vi "ExcelLoop.vi"() -> ()   [LabVIEW 2017]
uses:
  <vilib>/Utility/file.llb/Read Delimited Spreadsheet (DBL).vi
panel:
  in  "disabled index (row) 3":i32
  in  "disabled index (row) 2":i32
  in  "disabled index (row)":i32
  out "Time":i32
  out "Numeric 6":i32
  out "Numeric 5":i32
  out "Numeric 4":i32
  out "Z Position":i32
  out "X Position":i32
  out "Y Position":i32
  out "Speed Z":i32
  out "Speed X":i32
  out "Speed Y":i32
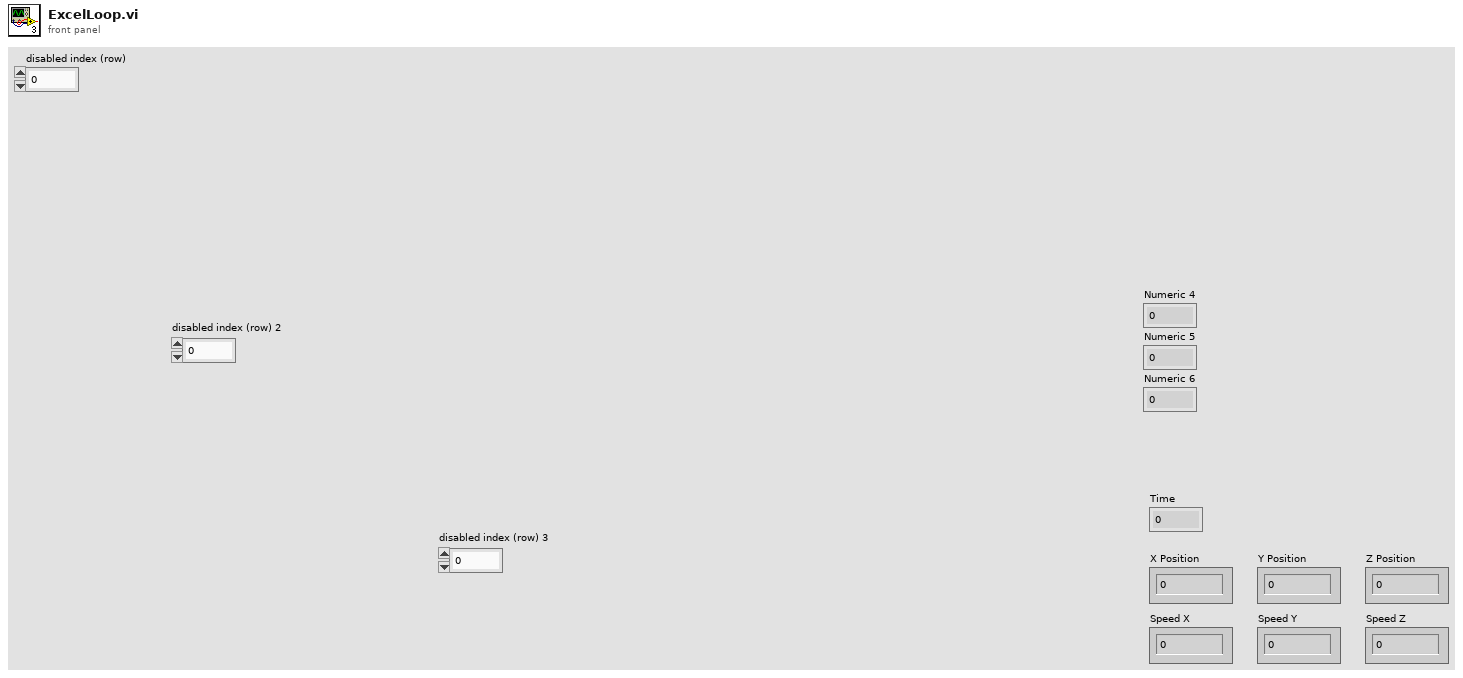
[diagram p1: front panel]
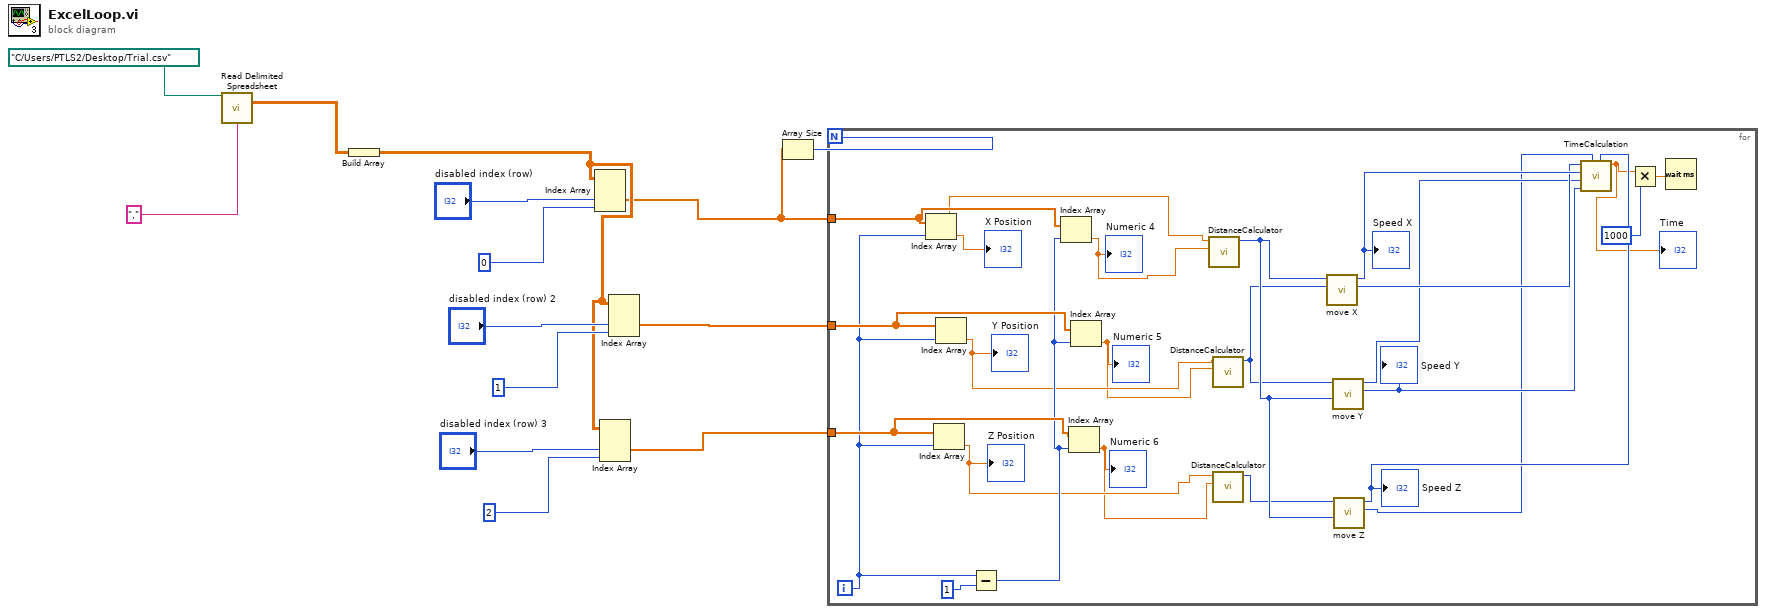
[diagram p0: block diagram]
diagram:
  n1 = call-poly <vilib>:"Read Delimited Spreadsheet.vi"("file path (dialog if empty)"=path "C:/Users/PTLS2/Desktop/Trial.csv", "delimiter (\\t)"="," ("delimiter (\\t)")) -> ("all rows"=w11:dbl[][])  [unwired: 8 in, 5 out]
  n2 = Build Array(w11) -> (w4:dbl[][][])
  n3 = Index Array(array=w4, index (dim 1)="disabled index (row)", index (dim 2)=0 ("disabled index (col)")) -> (element=w3:dbl[])  [unwired: 1 in]
  n4 = Index Array(array=w4, index (dim 1)="disabled index (row) 3", index (dim 2)=2 ("disabled index (col)")) -> (element=w1:dbl[])  [unwired: 1 in]
  n5 = Index Array(array=w4, index (dim 1)="disabled index (row) 2", index (dim 2)=1 ("disabled index (col)")) -> (element=w2:dbl[])  [unwired: 1 in]
  n6 = Array Size(array=w3) -> (size(s)=w14:i32)
  n7 = for {
    N: w14 -> [_]
    tunnel: w3 -> [w30]
    tunnel: w2 -> [w31]
    tunnel: w1 -> [w32]
    i -> [w24]
    n8 = Index Array(array=w30, index=w24) -> (element=w23:dbl)
    "X Position" <- w23
    n9 = Index Array(array=w32, index=w24) -> (element=w18:dbl)
    "Z Position" <- w18
    n10 = Index Array(array=w31, index=w24) -> (element=w20:dbl)
    "Y Position" <- w20
    n11 = Subtract(x=w24, y=1) -> (x-y=w25:i32)
    n12 = Index Array(array=w30, index=w25) -> (element=w22:dbl)
    "Numeric 4" <- w22
    n13 = Index Array(array=w32, index=w25) -> (element=w17:dbl)
    "Numeric 6" <- w17
    n14 = Index Array(array=w31, index=w25) -> (element=w19:dbl)
    "Numeric 5" <- w19
    n15 = call "DistanceCalculator.vi"("Number2"=w22, "Number1"=w23) -> ("Distance"=w21:i32)  [unwired: 9 in]
    n16 = call "DistanceCalculator.vi"("Number2"=w19, "Number1"=w20) -> ("Distance"=w15:i32)  [unwired: 9 in]
    n17 = call "DistanceCalculator.vi"("Number2"=w17, "Number1"=w18) -> ("Distance"=w16:i32)  [unwired: 9 in]
    n18 = call "move X.vi"("y mm"=w15, "x mm"=w21) -> ("X Position"=w37:i32, "Speed X"=w38:i32)  [unwired: 8 in]
    "Speed X" <- w38
    n19 = call "move Y.vi"("x mm"=w21, "y mm"=w15) -> ("Y Speed"=w35:i32, "Y Position"=w36:i32)  [unwired: 8 in]
    "Speed Y" <- w35
    n20 = call "move Z.vi"("x mm"=w21, "z mm"=w16) -> ("Z Position"=w33:i32, "Z Speed"=w34:i32)  [unwired: 8 in]
    "Speed Z" <- w34
    n21 = call "TimeCalculation.vi"("Speed Z"=w34, "Position Z"=w33, "SpeedY"=w35, "Y Position"=w36, "Speed X"=w38, "X Position"=w37) -> ("Time"=w27:dbl)  [unwired: 5 in]
    "Time" <- w27
    n22 = Multiply(x=w27, y=1000) -> (x*y=w29:dbl)
    n23 = Wait (ms)(milliseconds to wait=w29) -> ()  [unwired: 1 out]
  }
